vi "IBM4_PWM.vi"(8 "error in":errorcluster, 9 "PWM(%)":dbl=50.0, 10 "Pin#":i32=9, 11 "COM resource in":refnum<visa-resource-name>="COM9") -> (0 "error out":errorcluster, 3 "COM resource out":refnum<visa-resource-name>="COM9")   [LabVIEW 2021, in "IBM4.lvlib"]
doc: "This VI interfaces with the IBM4 to set a pulse wave modulated (PWM) output signal.\nThe output Pin# must be: 5,7,9,10-13.\nThe PWM output must be between 0 and 100, and is a floating point value."
uses:
  <instrlib>/IBM4/IBM4.lvlib
panel:
  out "read buffer":string="PWMset 13 = 10.0 \r\n"
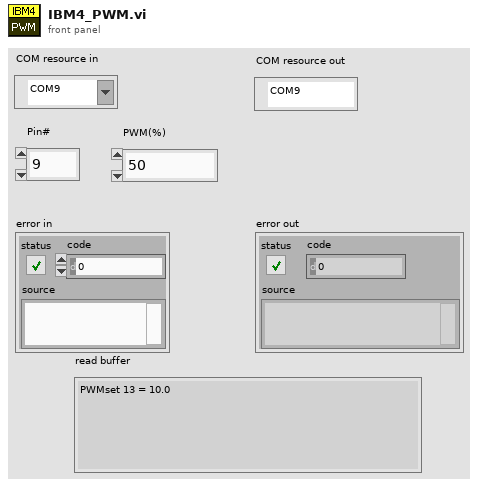
[diagram p1: front panel]
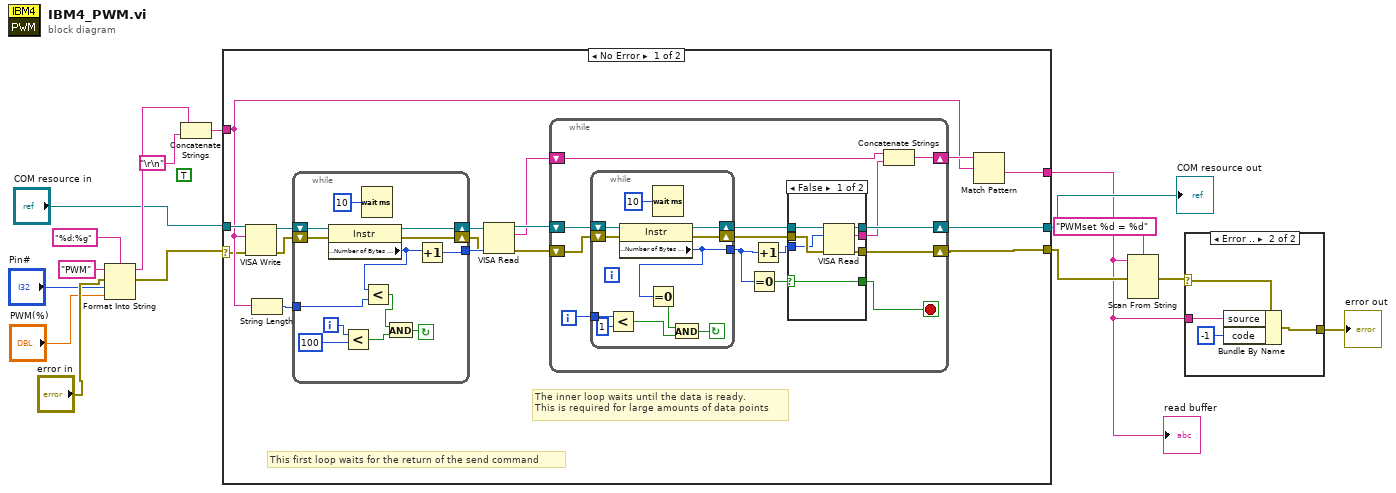
[diagram p0: block diagram]
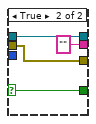
[diagram p3: hidden frame]
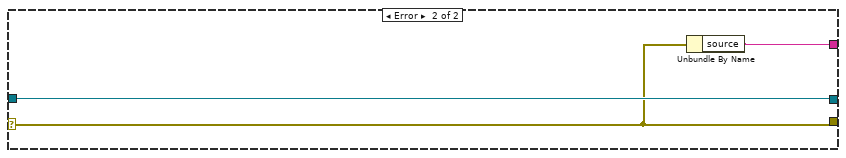
[diagram p4: hidden frame]
diagram:
  (unwired) TRUE ("Enable Termination\nChar (T)")
  n1 = Format Into String(format string="%d:%g", initial string="PWM", error in="error in", "Pin#", "PWM(%)") -> (resulting string=w7:string, error out=w1:errorcluster)
  n2 = Concatenate Strings(w7, "\r\n") -> (w6:string)
  n3 = case shown="No Error" w1 {
    selector: w1 -> [w19 w82]
    tunnel: "COM resource in" -> [w32 w84]
    tunnel: [w18 w82] -> w10
    tunnel: [w30 w83] -> w3
    tunnel: w6 -> [w29 _]
    tunnel: [w17 w84] -> w11
    frame No Error {
      # "The inner loop waits until the data is ready.\nThis is required for large amounts of data points"
      # "This first loop waits for the return of the send command"
      n4 = VISA Write(VISA resource name=w32, write buffer=w29, error in (no error)=w19) -> (VISA resource name out=w28:refnum<visa-resource-name>, error out=w27:errorcluster)  [unwired: 1 out]
      n5 = String Length(string=w29) -> (length=w20:i32)
      n6 = while {
        tunnel: [w34] -> w25
        shift-right: [w44] -> w26
        shift-left: w28 -> [w45]
        shift-right: [w42] -> w24
        shift-left: w27 -> [w43]
        tunnel: w20 -> [w40]
        i -> [w35]
        stop <- w38 continue-if-true
        n7 = property class="Instr"(reference=w45, error in=w43) -> (reference out=w44:refnum<visa-resource-name>, error out=w42:errorcluster, "Serial Settings:Number of Bytes at Serial Port"=w33:u32)
        n8 = Less?(x=w35, y=100) -> (x < y?=w37:bool)
        n9 = Wait (ms)(milliseconds to wait=u32 10) -> ()  [unwired: 1 out]
        n10 = Less?(x=w33, y=w40) -> (x < y?=w36:bool)
        n11 = And(x=w36, y=w37) -> (x .and. y?=w38:bool)
        n12 = Increment(x=w33) -> (x+1=w34:u32)
      }
      n13 = VISA Read(VISA resource name=w26, byte count=w25, error in (no error)=w24) -> (VISA resource name out=w23:refnum<visa-resource-name>, read buffer=w21:string, error out=w22:errorcluster)  [unwired: 1 out]
      n14 = while {
        shift-right: [w59] -> w17
        shift-left: w23 -> [w57]
        shift-right: [w58] -> w18
        shift-left: w22 -> [w55]
        shift-right: [w53] -> w31
        shift-left: w21 -> [w51]
        i -> [w50]
        stop <- w46 stop-if-true
        n15 = while {
          tunnel: [w76] -> w49
          shift-right: [w80] -> w56
          shift-left: w57 -> [w81]
          shift-right: [w78] -> w54
          shift-left: w55 -> [w79]
          tunnel: w50 -> [w75]
          stop <- w73 continue-if-true
          n16 = Less?(x=w75, y=1) -> (x < y?=w72:bool)
          n17 = property class="Instr"(reference=w81, error in=w79) -> (reference out=w80:refnum<visa-resource-name>, error out=w78:errorcluster, "Serial Settings:Number of Bytes at Serial Port"=w76:u32)
          n18 = Equal To 0?(x=w76) -> (x = 0?=w71:bool)
          n19 = Wait (ms)(milliseconds to wait=u32 10) -> ()  [unwired: 1 out]
          n20 = And(x=w71, y=w72) -> (x .and. y?=w73:bool)
        }
        n21 = Equal To 0?(x=w49) -> (x = 0?=w47:bool)
        n22 = Increment(x=w49) -> (x+1=w48:u32)
        n23 = case shown="False" w47 {
          selector: w47 -> [w60 w69]
          tunnel: [w66 w70] -> w59
          tunnel: [w65 w68] -> w58
          tunnel: w56 -> [w64 w70]
          tunnel: w54 -> [w63 w68]
          tunnel: [w62 "" ("read buffer")] -> w52
          tunnel: w48 -> [w61 _]
          tunnel: [w60 w69] -> w46
          frame False {
            n24 = VISA Read(VISA resource name=w64, byte count=w61, error in (no error)=w63) -> (VISA resource name out=w66:refnum<visa-resource-name>, read buffer=w62:string, error out=w65:errorcluster)  [unwired: 1 out]
          }
          frame True {
          }
        }
        n25 = Concatenate Strings(w51, w52) -> (w53:string)
      }
      n26 = Match Pattern(string=w31, regular expression=w29) -> (after substring=w30:string)  [unwired: 1 in, 3 out]
    }
    frame Error {
      n27 = Unbundle By Name(w82) -> ("source"=w83:string)
    }
  }
  "COM resource out" <- w11
  "read buffer" <- w3
  n28 = Scan From String(format string="PWMset %d = %d", input string=w3, error in=w10) -> (error out=w5:errorcluster)  [unwired: 5 in, 2 out]
  n29 = case shown="Error .." w5 {
    selector: w5 -> [w85 w89]
    tunnel: [w85 w87] -> w4
    tunnel: w3 -> [_ w88]
    frame No Error {
    }
    frame Error {
      n30 = Bundle By Name(cluster=w89, "source"=w88, "code"=-1) -> (w87:errorcluster)
    }
  }
  "error out" <- w4
